vi "TSM SSC Digital Configure Voltage Levels.vi"(0 "Digital TSM In":T1, 1 "vol (V)":dbl format="%#_6p", 2 "voh (V)":dbl format="%#_6p", 5 "vih (V)":dbl format="%#_6p", 7 "vil (V)":dbl format="%#_6p", 9 "vterm (V)":dbl format="%#_6p", 11 "error in":errorcluster) -> (4 "Digital TSM Out":T1, 15 "error out":errorcluster)   [LabVIEW 2020]
doc: "Configures voltage levels for the specified pin(s) and pin group(s)."
uses:
  TSM/TSM SSC Digital.ctl
  <vilib>/NI_TestStand_SemiconductorModule/NI_TestStand_Semiconductor_Module.lvlibp/PinMap/Digital Pattern/PinQueryContext/DigitalPatternPinQueryContext.lvclass
  SSC Digital/SSC Digital.ctl
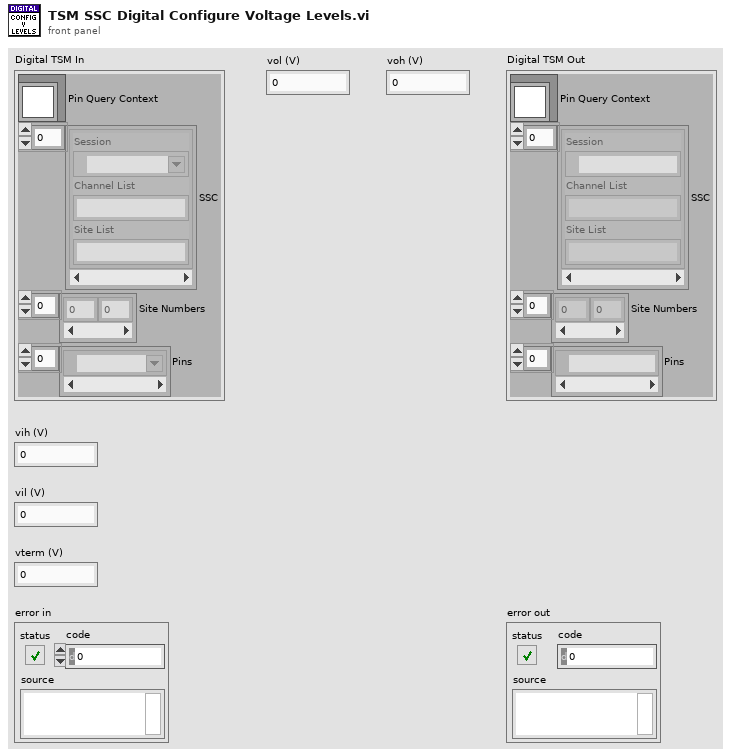
[diagram p1: front panel]
types:
  T1 = typedef "TSM SSC Digital.ctl" = cluster{"Pin Query Context":refnum<class "DigitalPatternPinQueryContext.lvclass">, "SSC":T2[], "Site Numbers":i32[], "Pins":tag[]}
  T2 = typedef "SSC Digital.ctl" = cluster{"Session":refnum<k15>, "Channel List":string, "Site List":string}
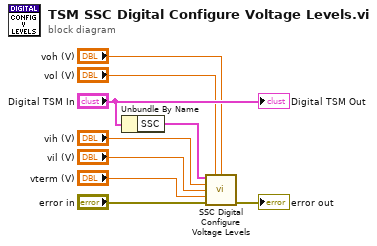
[diagram p0: block diagram]
diagram:
  n1 = Unbundle By Name("Digital TSM In") -> ("SSC"=w8:T2[])
  n2 = call "SSC Digital Configure Voltage Levels.vi"("Digital SSC in"=w8, "vol (V)"="vol (V)", "voh (V)"="voh (V)", "vih (V)"="vih (V)", "vil (V)"="vil (V)", "vterm (V)"="vterm (V)", "error in"="error in") -> ("error out"=→"error out":errorcluster)  [unwired: 7 in, 1 out]
  "Digital TSM Out" <- "Digital TSM In"
